vi "Actor Core.vi"(8 "error in":errorcluster, 11 "Stepper in":refnum<class "Stepper.lvclass">) -> (0 "error out":errorcluster, 3 "Actor out":refnum<class "Actor.lvclass">)   [LabVIEW 2015, in "Stepper.lvclass"]
doc: "(<B>Filename</B>: Actor Framework.lvlib:Actor.lvclass:Actor Core.vi)\n\nReceives messages to the actor, reacts to them, and initiates any error handling that may shut the actor down.\n\nDescendant classes may override this VI to append parallel tasks for the actor to complete while it handles messages. Overrides use the Call Parent Method node."
uses:
  Stepper.lvclass
  <vilib>/ActorFramework/Actor/Actor.lvclass
  Controls/Syringe State Enumerator.ctl
  Stepper.lvclass/Stepper.ctl
  CO2 Actor/CO2 Actor.lvclass
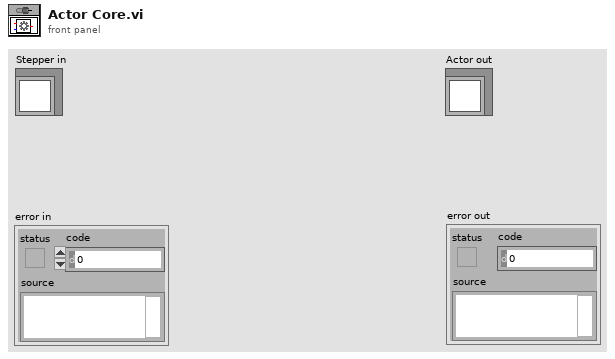
[diagram p1: front panel]
types:
  T1 = typedef "Syringe State Enumerator.ctl" = enum16{"Initialize", "Standby", "Enable", "Idle", "Prepare for Run", "Run", "Home", "Disable"}
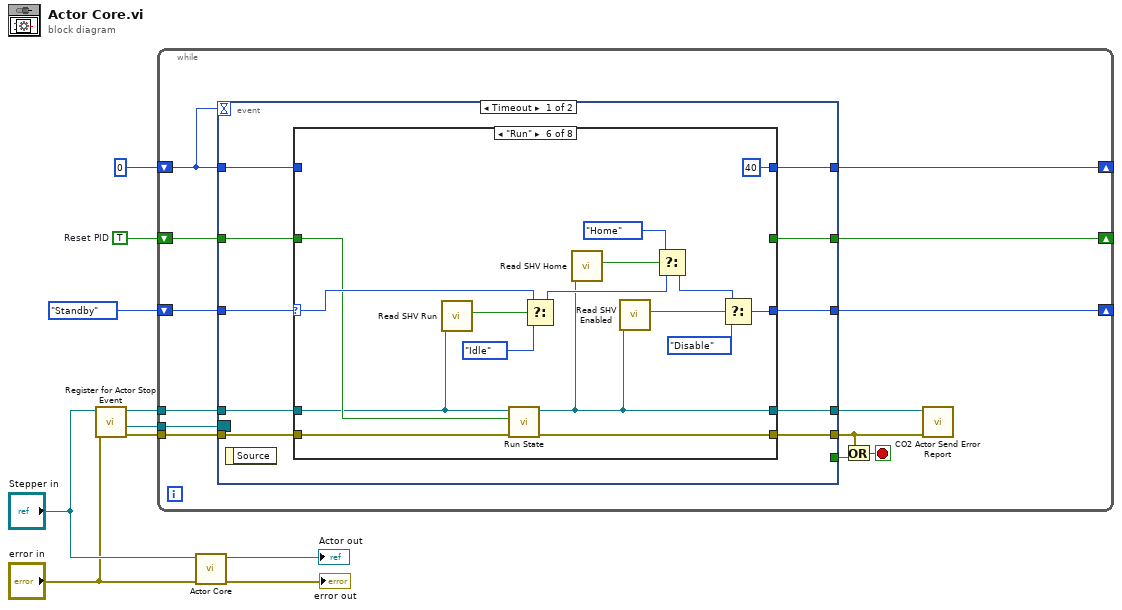
[diagram p0: block diagram]
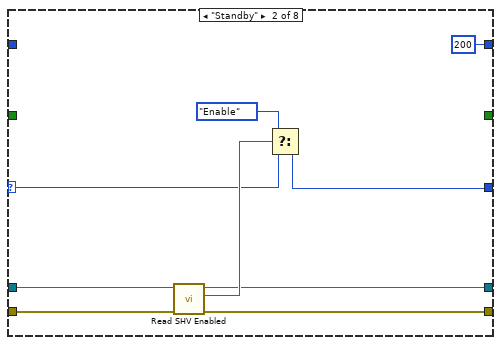
[diagram p3: hidden frame]
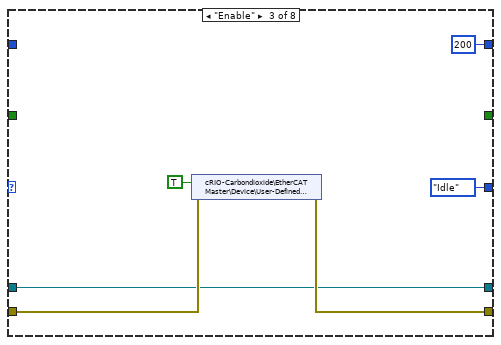
[diagram p4: hidden frame]
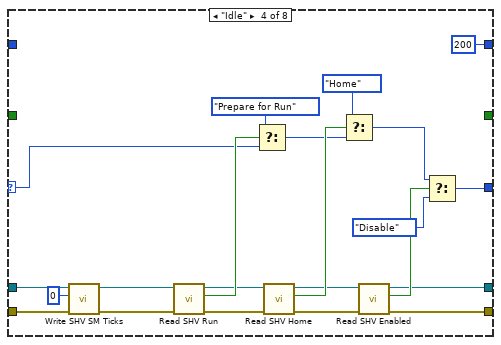
[diagram p5: hidden frame]
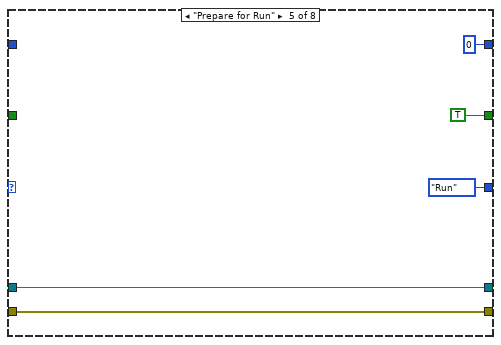
[diagram p6: hidden frame]
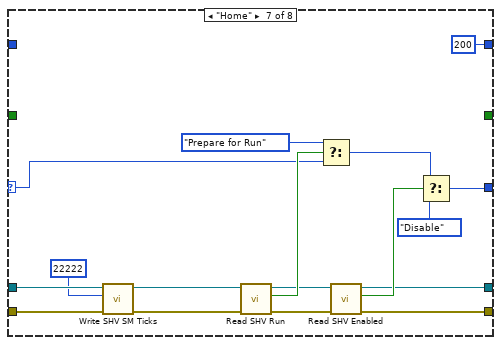
[diagram p7: hidden frame]
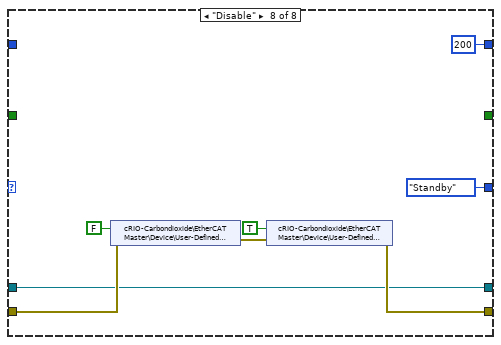
[diagram p8: hidden frame]
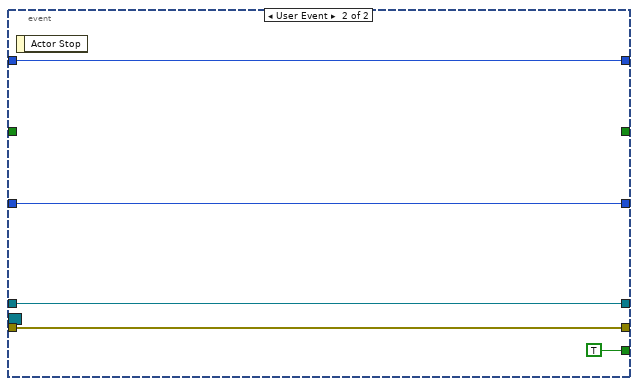
[diagram p9: hidden frame]
diagram:
  w1 = TRUE  # Reset PID
  n1 = call "Register for Actor Stop Event.vi"("error in (no error)"="error in", "CO2 Actor in"="Stepper in") -> ("error out"=w6:errorcluster, "Event Registration Refnum"=w4:refnum<event-registration>, "CO2 Actor out"=w5:refnum<class "Stepper.lvclass">)  [unwired: 7 in]
  n2 = while {
    tunnel: w6 -> [w22]
    tunnel: w5 -> [w21]
    tunnel: w4 -> [w23]
    shift-right: [w17] -> _
    shift-left: 0 -> [w18]
    shift-right: [w15] -> _
    shift-left: Syringe_State_Enumerator."Standby" -> [w16]
    shift-right: [w14] -> _
    shift-left: w1 -> [w13]
    stop <- w19 stop-if-true
    n3 = event shown="[0] Timeout" {
      selector: w23 -> [_ _]
      dyn-events: _ -> [_ _]
      timeout: w18 -> [_ _]
      tunnel: w22 -> [w32 w125]
      tunnel: [w29 w125] -> w11
      tunnel: w21 -> [w33 w124]
      tunnel: [w30 w124] -> w12
      tunnel: [_ TRUE] -> w20
      tunnel: w18 -> [w27 w122]
      tunnel: [w26 w122] -> w17
      tunnel: w16 -> [w31 w121]
      tunnel: [w28 w121] -> w15
      tunnel: [w25 _] -> w14
      tunnel: w13 -> [w24 _]
      event Timeout {
        n4 = event-data() -> ()  [unwired: 1 in, 1 out]
        n5 = case shown="\"Run\"" w31 {
          selector: w31 -> [w37 w45 _ w62 _ w85 w106 _]
          tunnel: w33 -> [w35 w39 w49 w65 w76 w80 w103 w114]
          tunnel: w32 -> [w36 w40 w51 w61 w75 w95 w102 w117]
          tunnel: [w35 w38 w49 w58 w76 w81 w100 w114] -> w30
          tunnel: [w36 w41 w50 w66 w75 w94 w105 w116] -> w29
          tunnel: [w37 w44 Syringe_State_Enumerator."Idle" w64 Syringe_State_Enumerator."Run" ("f") w84 w108 Syringe_State_Enumerator."Standby" ("f")] -> w28
          tunnel: w27 -> [w34 _ _ _ _ _ _ _]
          tunnel: [w34 200 200 200 0 40 200 200] -> w26
          tunnel: [_ _ _ _ TRUE _ _ _] -> w25
          tunnel: w24 -> [_ _ _ _ _ w82 _ _]
          frame "Initialize", Default {
          }
          frame "Standby" {
            n6 = call "Read SHV Enabled.vi"("error in (no error)"=w40, "Stepper in"=w39) -> ("error out"=w41:errorcluster, "data out"=w46:bool, "Stepper out"=w38:refnum<class "Stepper.lvclass">)  [unwired: 7 in]
            n7 = Select(t=Syringe_State_Enumerator."Enable", s=w46, f=w45) -> (s? t:f=w44:T1)
          }
          frame "Enable" {
            n8 = shared-variable "cRIO-Carbondioxide\\EtherCAT Master\\Device\\User-Defined Variables\\SM Enable Drive"(TRUE ("Enable Drive"), error in=w51) -> (error out=w50:errorcluster)
          }
          frame "Idle" {
            n9 = call "Write SHV SM Ticks.vi"("error in (no error)"=w61, "Ticks (0)"=i16 0 ("Ticks"), "Stepper in"=w65) -> ("error out"=w55:errorcluster, "Stepper out"=w54:refnum<class "Stepper.lvclass">)  [unwired: 7 in]
            n10 = call "Read SHV Run.vi"("error in (no error)"=w55, "Stepper in"=w54) -> ("error out"=w56:errorcluster, "data out"=w71:bool, "Stepper out"=w53:refnum<class "Stepper.lvclass">)  [unwired: 7 in]
            n11 = Select(t=Syringe_State_Enumerator."Prepare for Run", s=w71, f=w62) -> (s? t:f=w70:T1)
            n12 = call "Read SHV Home.vi"("error in (no error)"=w56, "Stepper in"=w53) -> ("error out"=w59:errorcluster, "data out"=w74:bool, "Stepper out"=w57:refnum<class "Stepper.lvclass">)  [unwired: 7 in]
            n13 = Select(t=Syringe_State_Enumerator."Home", s=w74, f=w70) -> (s? t:f=w69:T1)
            n14 = call "Read SHV Enabled.vi"("error in (no error)"=w59, "Stepper in"=w57) -> ("error out"=w66:errorcluster, "data out"=w68:bool, "Stepper out"=w58:refnum<class "Stepper.lvclass">)  [unwired: 7 in]
            n15 = Select(t=w69, s=w68, f=Syringe_State_Enumerator."Disable") -> (s? t:f=w64:T1)
          }
          frame "Prepare for Run" {
          }
          frame "Run" {
            n16 = call "Read SHV Run.vi"("Stepper in"=w80) -> ("data out"=w93:bool)  [unwired: 8 in, 2 out]
            n17 = call "Run State.vi"("error in (no error)"=w95, "Reset"=w82, "Stepper in"=w80) -> ("error out"=w94:errorcluster, "Stepper out"=w81:refnum<class "Stepper.lvclass">)  [unwired: 7 in]
            n18 = Select(t=w85, s=w93, f=Syringe_State_Enumerator."Idle") -> (s? t:f=w88:T1)
            n19 = call "Read SHV Home.vi"("Stepper in"=w81) -> ("data out"=w91:bool)  [unwired: 8 in, 2 out]
            n20 = call "Read SHV Enabled.vi"("Stepper in"=w81) -> ("data out"=w89:bool)  [unwired: 8 in, 2 out]
            n21 = Select(t=Syringe_State_Enumerator."Home", s=w91, f=w88) -> (s? t:f=w87:T1)
            n22 = Select(t=w87, s=w89, f=Syringe_State_Enumerator."Disable") -> (s? t:f=w84:T1)
          }
          frame "Home" {
            n23 = call "Write SHV SM Ticks.vi"("error in (no error)"=w102, "Ticks (0)"=i16 22222 ("Ticks"), "Stepper in"=w103) -> ("error out"=w96:errorcluster, "Stepper out"=w98:refnum<class "Stepper.lvclass">)  [unwired: 7 in]
            n24 = call "Read SHV Run.vi"("error in (no error)"=w96, "Stepper in"=w98) -> ("error out"=w99:errorcluster, "data out"=w109:bool, "Stepper out"=w97:refnum<class "Stepper.lvclass">)  [unwired: 7 in]
            n25 = Select(t=Syringe_State_Enumerator."Prepare for Run", s=w109, f=w106) -> (s? t:f=w104:T1)
            n26 = call "Read SHV Enabled.vi"("error in (no error)"=w99, "Stepper in"=w97) -> ("error out"=w105:errorcluster, "data out"=w112:bool, "Stepper out"=w100:refnum<class "Stepper.lvclass">)  [unwired: 7 in]
            n27 = Select(t=w104, s=w112, f=Syringe_State_Enumerator."Disable") -> (s? t:f=w108:T1)
          }
          frame "Disable" {
            n28 = shared-variable "cRIO-Carbondioxide\\EtherCAT Master\\Device\\User-Defined Variables\\SM Enable Drive"(FALSE ("Enable Drive"), error in=w117) -> (error out=w115:errorcluster)
            n29 = shared-variable "cRIO-Carbondioxide\\EtherCAT Master\\Device\\User-Defined Variables\\SM Clear Faults"(TRUE ("Clear Faults"), error in=w115) -> (error out=w116:errorcluster)
          }
        }
      }
      event User Event {
        n30 = event-data() -> ()  [unwired: 1 in, 1 out]
      }
    }
    n31 = Or(x=w11, y=w20) -> (x .or. y?=w19:bool)
    n32 = call-dynamic "CO2 Actor Send Error Report.vi"("Error From Sender"=w11, "CO2 Actor in"=w12) -> ()  [unwired: 9 in, 1 out]
  }
  n33 = call-parent "Actor Core.vi"("error in"="error in", "CO2 Actor in"="Stepper in") -> ("error out"=→"error out":errorcluster, "Actor out"=→"Actor out":refnum<class "Actor.lvclass">)  [unwired: 8 in]
